vi "LCD(SubVI).vi"(11 "String":string) -> ()   [LabVIEW 2017]
uses:
  <vilib>/myRIO/Instrument Drivers/Onboard IO/UART/typedef/VISA Configuration.ctl
  <vilib>/Instr/_visa.llb/VISA Configure Serial Port (Instr).vi
  <vilib>/myRIO/Express VI/Onboard IO/UART/UART Express VI.xnode
  <vilib>/myRIO/Instrument Drivers/Onboard IO/UART/UART.lvlib
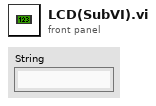
[diagram p1: front panel]
types:
  T1 = typedef "UART.lvlib/VISA Configuration.ctl" = cluster{"baud rate (9600)":u32, "data bits (8)":u16, "parity (0:none)":enum16{"None", "Odd", "Even", "Mark", "Space"}, "stop bits (10: 1 bit)":u16, "flow control (0:none)":u16, "termination char\n(0xA = '\\n' = LF) ":u8, "Enable Termination\nChar (T)":bool, "timeout (10sec)":u32}
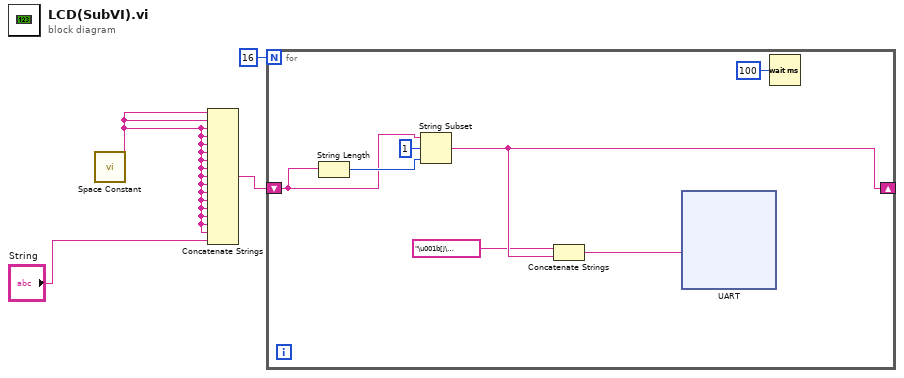
[diagram p0: block diagram]
diagram:
  n1 = call <vilib>:"Space Constant.vi"() -> ("String"=w2:string)
  n2 = Concatenate Strings(w2, w2, w2, w2, w2, w2, w2, w2, w2, w2, w2, w2, w2, w2, w2, w2, "String") -> (w3:string)
  n3 = for {
    N: 16 -> [_]
    shift-right: [w8] -> _
    shift-left: w3 -> [w9]
    n4 = String Length(string=w9) -> (length=w11:i32)
    n5 = String Subset(string=w9, offset (0)=1, length (rest)=w11) -> (substring=w8:string)
    n6 = Concatenate Strings("\u001b[j\u001b[1h" ("string"), w8) -> (w6:string)
    n7 = xnode "UART"("Characters to Write"=w6) -> ()  [unwired: 1 in, 2 out]
    n8 = Wait (ms)(milliseconds to wait=u32 100) -> ()  [unwired: 1 out]
  }
